vi "Process Move.vi"(9 "Direction":T1, 10 "Action":T2, 11 "Base Builder In":refnum<class "Formics.lvclass">) -> (3 "Base Builder Out":refnum<class "Formics.lvclass">)   [LabVIEW 2015, in "Formics.lvclass"]
uses:
  Formics.lvclass
  Type Defs/Action Enum.ctl
  Type Defs/Direction Enum.ctl
  Formics.lvclass/Formics.ctl
  SubVIs/Read-Only Globals.vi
  Square/Square.lvclass
  Type Defs/SB Type Defs.lvlib
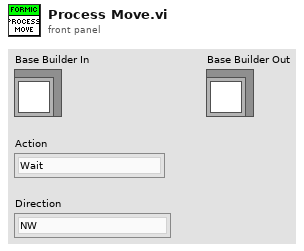
[diagram p1: front panel]
types:
  T1 = typedef "SB Type Defs.lvlib/Direction Enum.ctl" = enum16{"NW", "N", "NE", "E", "SE", "S", "SW", "W"}
  T2 = typedef "SB Type Defs.lvlib/Action Enum.ctl" = enum16{"Wait", "Move", "Attack", "Replicate"}
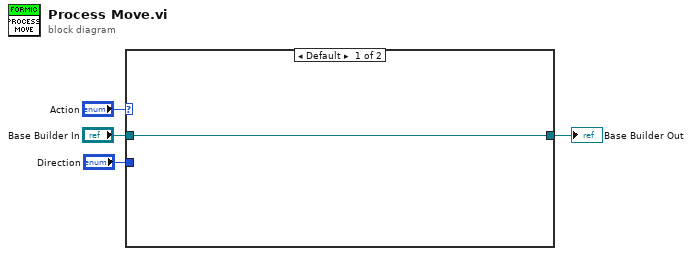
[diagram p0: block diagram]
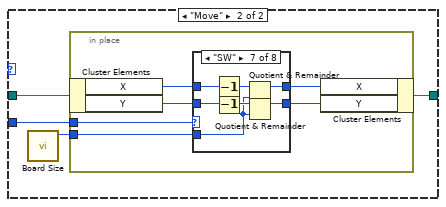
[diagram p2: hidden frame]
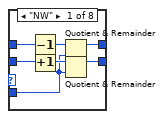
[diagram p3: hidden frame]
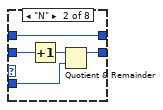
[diagram p4: hidden frame]
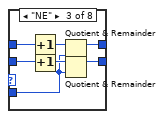
[diagram p5: hidden frame]
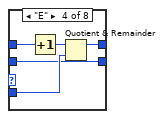
[diagram p6: hidden frame]
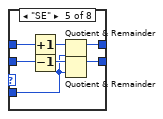
[diagram p7: hidden frame]
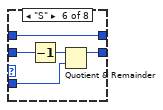
[diagram p8: hidden frame]
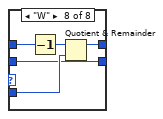
[diagram p9: hidden frame]
diagram:
  n1 = case shown="Default" "Action" {
    tunnel: "Base Builder In" -> [w5 w9]
    tunnel: [w5 w6] -> w2
    tunnel: "Direction" -> [_ w8]
    frame Default {
    }
    frame "Move" {
      n2 = call "Board Size.vi"() -> ("Board Size"=w7:i32)  [unwired: 11 in]
      n3 = in-place {
        in-place-border: w8 -> [w15]
        in-place-border: w7 -> [w12]
        n4 = in-place-cluster #1(w9) -> ("X"=w14:i32, "Y"=w13:i32)
        n5 = case shown="\"SW\"" w15 {
          tunnel: w14 -> [w21 w23 w33 w39 w45 w47 w57 w63]
          tunnel: w13 -> [w22 w27 w34 w35 w46 w51 w58 w59]
          tunnel: [w19 w25 w31 w35 w43 w49 w55 w59] -> w11
          tunnel: [w16 w23 w28 w36 w40 w47 w52 w60] -> w10
          tunnel: w12 -> [w17 w24 w29 w37 w41 w48 w53 w61]
          frame "NW" {
            n6 = Decrement(x=w21) -> (x-1=w18:i32)
            n7 = Increment(x=w22) -> (x+1=w20:i32)
            n8 = Quotient & Remainder(x=w18, y=w17) -> (x-y*floor(x/y)=w16:i32)  [unwired: 1 out]
            n9 = Quotient & Remainder(x=w20, y=w17) -> (x-y*floor(x/y)=w19:i32)  [unwired: 1 out]
          }
          frame "N" {
            n10 = Increment(x=w27) -> (x+1=w26:i32)
            n11 = Quotient & Remainder(x=w26, y=w24) -> (x-y*floor(x/y)=w25:i32)  [unwired: 1 out]
          }
          frame "NE" {
            n12 = Increment(x=w33) -> (x+1=w30:i32)
            n13 = Increment(x=w34) -> (x+1=w32:i32)
            n14 = Quotient & Remainder(x=w30, y=w29) -> (x-y*floor(x/y)=w28:i32)  [unwired: 1 out]
            n15 = Quotient & Remainder(x=w32, y=w29) -> (x-y*floor(x/y)=w31:i32)  [unwired: 1 out]
          }
          frame "E" {
            n16 = Increment(x=w39) -> (x+1=w38:i32)
            n17 = Quotient & Remainder(x=w38, y=w37) -> (x-y*floor(x/y)=w36:i32)  [unwired: 1 out]
          }
          frame "SE" {
            n18 = Increment(x=w45) -> (x+1=w42:i32)
            n19 = Decrement(x=w46) -> (x-1=w44:i32)
            n20 = Quotient & Remainder(x=w42, y=w41) -> (x-y*floor(x/y)=w40:i32)  [unwired: 1 out]
            n21 = Quotient & Remainder(x=w44, y=w41) -> (x-y*floor(x/y)=w43:i32)  [unwired: 1 out]
          }
          frame "S" {
            n22 = Decrement(x=w51) -> (x-1=w50:i32)
            n23 = Quotient & Remainder(x=w50, y=w48) -> (x-y*floor(x/y)=w49:i32)  [unwired: 1 out]
          }
          frame "SW" {
            n24 = Decrement(x=w57) -> (x-1=w54:i32)
            n25 = Decrement(x=w58) -> (x-1=w56:i32)
            n26 = Quotient & Remainder(x=w54, y=w53) -> (x-y*floor(x/y)=w52:i32)  [unwired: 1 out]
            n27 = Quotient & Remainder(x=w56, y=w53) -> (x-y*floor(x/y)=w55:i32)  [unwired: 1 out]
          }
          frame "W" {
            n28 = Decrement(x=w63) -> (x-1=w62:i32)
            n29 = Quotient & Remainder(x=w62, y=w61) -> (x-y*floor(x/y)=w60:i32)  [unwired: 1 out]
          }
        }
        n30 = in-place-cluster #1("X"=w10, "Y"=w11) -> (w6:refnum<class "Formics.lvclass">)
      }
    }
  }
  "Base Builder Out" <- w2
